vi "TF3710LibExample.vi"() -> ()   [LabVIEW 2020]
uses:
  <userlib>/Beckhoff-LabVIEW-Interface/_DependsOn/TypeDefs/Low-Levels/Symbol Interface Mode.ctl
  <userlib>/Beckhoff-LabVIEW-Interface/_DependsOn/With TypeResolving/Read Sync Single TypeResolved.vi
  <userlib>/Beckhoff-LabVIEW-Interface/_DependsOn/With TypeResolving/Read Async Single TypeResolved.vi
panel:
  out "Read Status? 8":bool
  out "Data 8":variant
  out "Read Status? 7":bool
  out "Data 7":variant
  out "Read Status? 6":bool
  out "Data 6":variant
  out "Read Status? 5":bool
  out "Data 5":variant
  out "Read Status? 4":bool
  out "Data 4":variant
  out "ReadGrpSymbols":string[](array[string])
  out "PortInfo":string
  out "error out":errorcluster
  in  "error in (no error)":errorcluster
  in  "Symbol file path":path=path "C:/MSDApps/GitHub-Projects/EDP Emotor/Anoop_LabviewTwincatADSTesting/ADS Read Symbols.xml"
  out "Read Status?":bool
  out "Read Status? 2":bool
  out "Read Status? 3":bool
  out "Data 1":variant
  out "Data 2":variant
  out "Data 3":variant
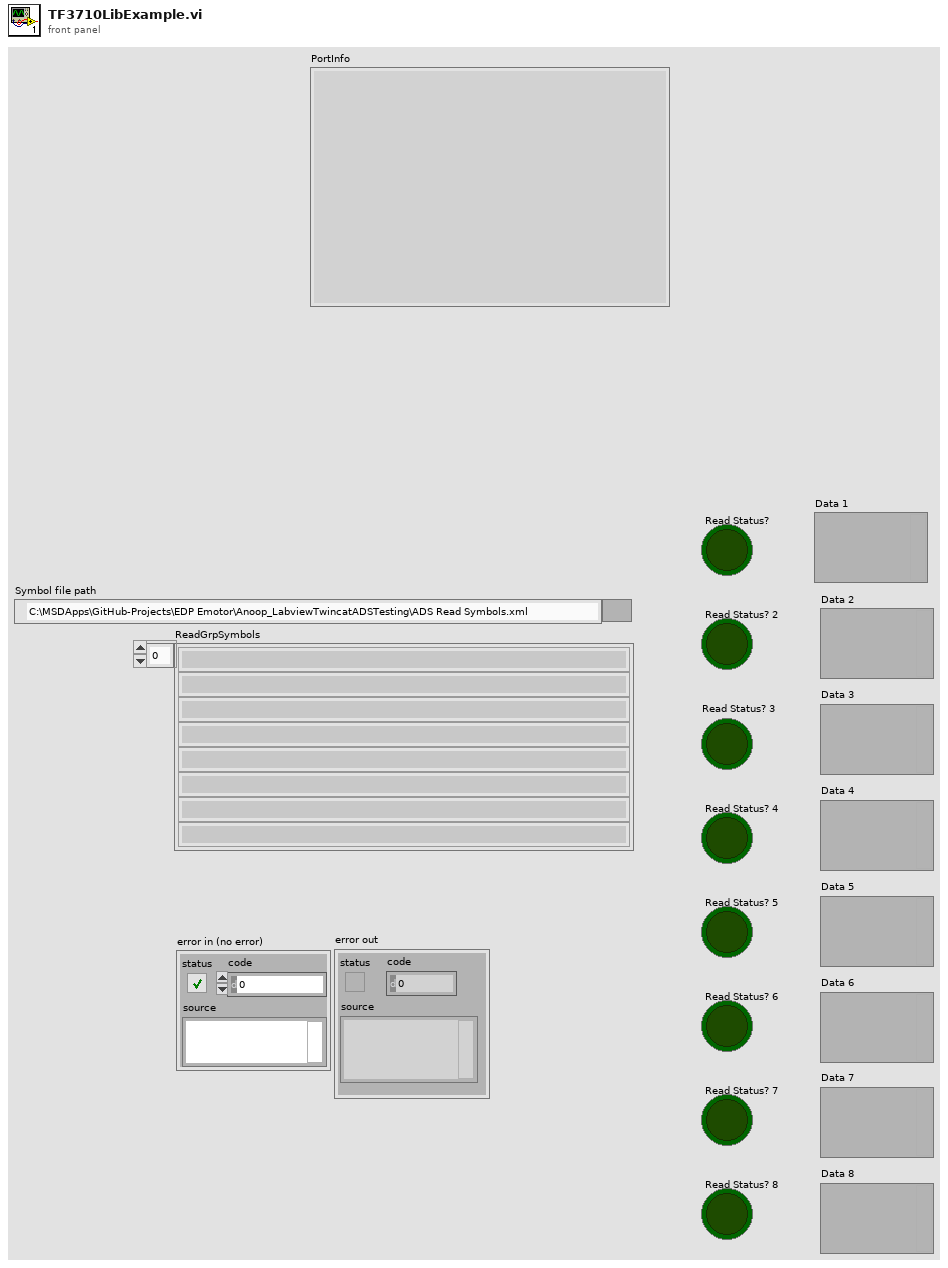
[diagram p1: front panel]
types:
  T1 = typedef "Symbol Interface Mode.ctl" = enum16{"Read Only", "Write Only", "Read & Write"}
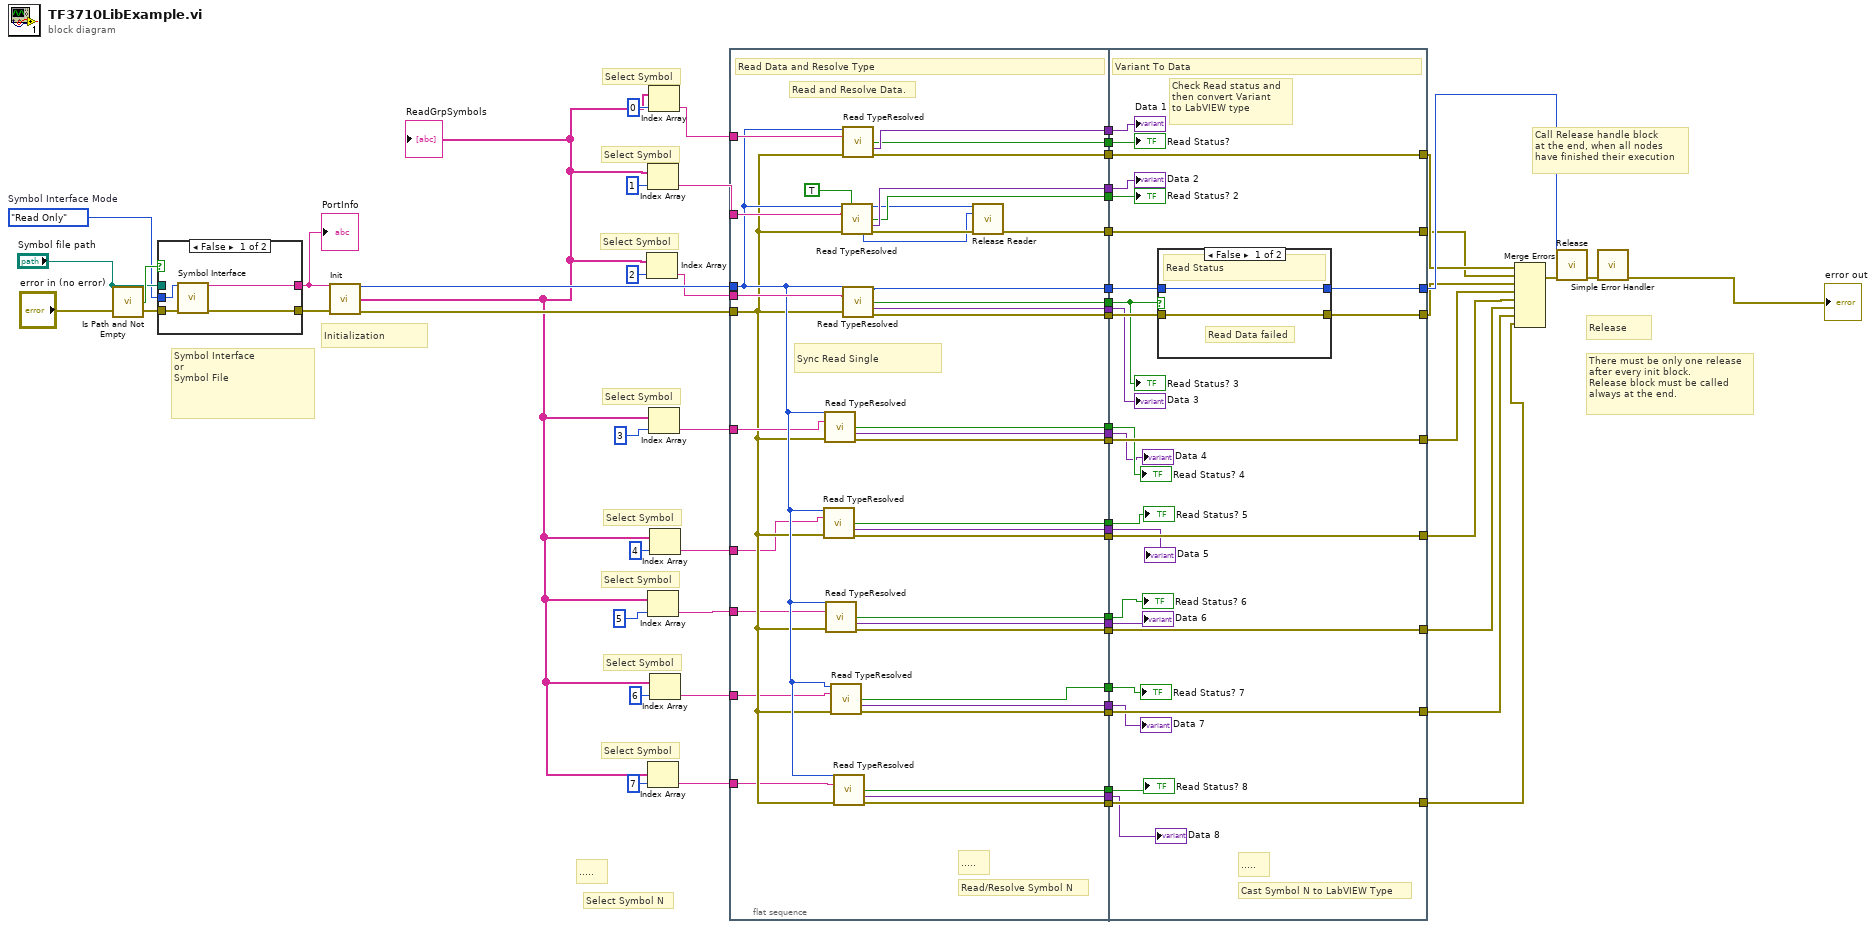
[diagram p0: block diagram]
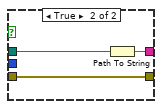
[diagram p2: hidden frame]
diagram:
  w36 = Symbol_Interface_Mode."Read Only"  # Symbol Interface Mode
  # "Select Symbol"
  # "Select Symbol"
  # "Select Symbol"
  # "Select Symbol"
  # "Select Symbol"
  # "Symbol Interface\nor\nSymbol File"
  # "Call Release handle block\nat the end, when all nodes\nhave finished their execution"
  # "Select Symbol N"
  # "....."
  # "Select Symbol"
  # "Select Symbol"
  # "There must be only one release\nafter every init block.\nRelease block must be called\nalways at the end."
  # "Select Symbol"
  # "Initialization"
  # "Release"
  n1 = call <vilib>:"Is Path and Not Empty.vi"("path"="Symbol file path") -> ("Is Path and Not Empty?"=w39:bool)  [unwired: 4 in]
  n2 = case shown="False" w39 {
    tunnel: [w66 w69] -> w32
    tunnel: "Symbol file path" -> [_ w68]
    tunnel: [w65 w67] -> w38
    tunnel: w36 -> [w64 _]
    tunnel: "error in (no error)" -> [w63 w67]
    frame False {
      n3 = call <userlib>:"Symbol Interface.vi"("Symbol Interface Mode"=w64, "error in (no error)"=w63) -> ("PortInfo"=w66:string, "error out"=w65:errorcluster)  [unwired: 12 in]
    }
    frame True {
      n4 = Path To String(path=w68) -> (string=w69:string)
    }
  }
  "PortInfo" <- w32
  n5 = call <userlib>:"Init.vi"("XMLDescription"=w32, "error in (no error)"=w38) -> ("Handle"=w45:u32, "ReadGrpSymbols"=w26:string[], "error out"=w46:errorcluster)  [unwired: 9 in, 2 out]
  "ReadGrpSymbols" <- w26
  n6 = Index Array(array=w26, index=2) -> (element=w44:string)
  n7 = Index Array(array=w26, index=1) -> (element=w48:string)
  n8 = Index Array(array=w26, index=5) -> (element=w4:string)
  n9 = Index Array(array=w26, index=7) -> (element=w2:string)
  n10 = Index Array(array=w26, index=0) -> (element=w47:string)
  n11 = Index Array(array=w26, index=3) -> (element=w25:string)
  n12 = Index Array(array=w26, index=4) -> (element=w5:string)
  n13 = Index Array(array=w26, index=6) -> (element=w3:string)
  n14 = flat-sequence {
    tunnel: w48 -> [w108]
    tunnel: w47 -> [w105]
    tunnel: w46 -> [w89]
    tunnel: w45 -> [w91]
    tunnel: w44 -> [w103]
    tunnel: [w94] -> w62
    tunnel: [w106] -> w61
    tunnel: [w104] -> w60
    tunnel: [w102] -> w59
    tunnel: [w101] -> w58
    tunnel: [w100] -> w57
    tunnel: [w99] -> w56
    tunnel: [w98] -> w55
    tunnel: [w97] -> w54
    tunnel: [w96] -> w53
    tunnel: w25 -> [w90]
    tunnel: [w88] -> w23
    tunnel: [w87] -> w21
    tunnel: [w86] -> w19
    tunnel: [w85] -> w17
    tunnel: [w84] -> w15
    tunnel: [w83] -> w14
    tunnel: [w82] -> w13
    tunnel: [w81] -> w12
    tunnel: [w80] -> w11
    tunnel: [w79] -> w10
    tunnel: [w78] -> w9
    tunnel: [w77] -> w8
    tunnel: [w76] -> w7
    tunnel: [w75] -> w6
    tunnel: w5 -> [w74]
    tunnel: w4 -> [w73]
    tunnel: w3 -> [w72]
    tunnel: w2 -> [w71]
    tunnel: [w70] -> w1
    tunnel: [w130] -> w43
    tunnel: [w132] -> w40
    tunnel: [w135] -> w41
    tunnel: w62 -> [w135]
    tunnel: w61 -> [w134]
    tunnel: w60 -> [w131]
    tunnel: w59 -> [w133]
    tunnel: w58 -> [w126]
    tunnel: w57 -> [w125]
    tunnel: w56 -> [w124]
    tunnel: [w134] -> w42
    tunnel: w55 -> [w127]
    tunnel: w54 -> [w129]
    tunnel: w53 -> [w128]
    tunnel: [w123] -> w24
    tunnel: w23 -> [w123]
    tunnel: [w122] -> w22
    tunnel: w21 -> [w122]
    tunnel: [w121] -> w20
    tunnel: w19 -> [w121]
    tunnel: [w120] -> w18
    tunnel: w17 -> [w120]
    tunnel: [w119] -> w16
    tunnel: w15 -> [w119]
    tunnel: w14 -> [w118]
    tunnel: w13 -> [w117]
    tunnel: w12 -> [w116]
    tunnel: w11 -> [w115]
    tunnel: w10 -> [w114]
    tunnel: w9 -> [w113]
    tunnel: w8 -> [w112]
    tunnel: w7 -> [w111]
    tunnel: w6 -> [w110]
    tunnel: w1 -> [w109]
    frame #0 {
      # "Read and Resolve Data."
      # "Read/Resolve Symbol N"
      # "....."
      # "Sync Read Single"
      # "Read Data and Resolve Type"
      n15 = call-poly <userlib>:"Read TypeResolved.vi"("Handle"=w91, "SymbolName"=w74, "error constant"=w89) -> ("Read Status?"=w82:bool, "RData"=w76:variant, "error out"=w87:errorcluster)  [unwired: 9 in, 1 out]
      n16 = call-poly <userlib>:"Read TypeResolved.vi"("Handle"=w91, "SymbolName"=w90, "error constant"=w89) -> ("Read Status?"=w83:bool, "RData"=w75:variant, "error out"=w88:errorcluster)  [unwired: 9 in, 1 out]
      n17 = call-poly <userlib>:"Read TypeResolved.vi"("Handle"=w91, "SymbolName"=w73, "error constant"=w89) -> ("Read Status?"=w81:bool, "RData"=w70:variant, "error out"=w86:errorcluster)  [unwired: 9 in, 1 out]
      n18 = call-poly <userlib>:"Read TypeResolved.vi"("Handle"=w91, "SymbolName"=w72, "error constant"=w89) -> ("Read Status?"=w80:bool, "RData"=w77:variant, "error out"=w85:errorcluster)  [unwired: 9 in, 1 out]
      n19 = call-poly <userlib>:"Read TypeResolved.vi"("Handle"=w91, "SymbolName"=w71, "error constant"=w89) -> ("Read Status?"=w79:bool, "RData"=w78:variant, "error out"=w84:errorcluster)  [unwired: 9 in, 1 out]
      n20 = call-poly <userlib>:"Read TypeResolved.vi"("Handle"=w91, "Wait?"=TRUE, "SymbolName"=w108, "error constant"=w89) -> ("Handle"=w93:u32, "Read Status?"=w96:bool, "RData"=w100:variant, "ReadHdl"=w92:u32, "error out"=w107:errorcluster)  [unwired: 6 in, 1 out]
      n21 = call-poly <userlib>:"Read TypeResolved.vi"("Handle"=w91, "SymbolName"=w105, "error constant"=w89) -> ("Read Status?"=w97:bool, "RData"=w101:variant, "error out"=w106:errorcluster)  [unwired: 9 in, 1 out]
      n22 = call-poly <userlib>:"Read TypeResolved.vi"("Handle"=w91, "SymbolName"=w103, "error constant"=w89) -> ("Handle"=w102:u32, "Read Status?"=w98:bool, "RData"=w99:variant, "error out"=w104:errorcluster)  [unwired: 9 in]
      n23 = call <userlib>:"Release Reader.vi"("Handle"=w93, "ReadHandle"=w92, "error in (no error)"=w107) -> ("error out"=w94:errorcluster)  [unwired: 11 in, 1 out]
    }
    frame #1 {
      # "Check Read status and\nthen convert Variant \nto LabVIEW type"
      # "Cast Symbol N to LabVIEW Type"
      # "....."
      # "Variant To Data"
      n24 = case shown="False" w127 {
        tunnel: w133 -> [w137 w138]
        tunnel: [w136 w139] -> w132
        tunnel: w131 -> [w136 w139]
        tunnel: [w137 w138] -> w130
        frame False {
          # "Read Data failed"
          # "Read Status"
        }
        frame True {
          # "User Code here"
          # "Variant to Data"
        }
      }
      "Read Status?" <- w129
      "Read Status? 2" <- w128
      "Read Status? 3" <- w127
      "Data 1" <- w126
      "Data 2" <- w125
      "Data 3" <- w124
      "Read Status? 4" <- w118
      "Data 4" <- w110
      "Read Status? 5" <- w117
      "Data 5" <- w111
      "Read Status? 6" <- w116
      "Data 6" <- w109
      "Read Status? 7" <- w115
      "Data 7" <- w112
      "Read Status? 8" <- w114
      "Data 8" <- w113
    }
  }
  n25 = Merge Errors(w42, w41, w40, w24, w22, w20, w18, w16) -> (w52:errorcluster)
  n26 = call <userlib>:"Release.vi"("Handle"=w43, "error in (no error)"=w52) -> ("error out"=w35:errorcluster)  [unwired: 13 in]
  n27 = call <vilib>:"Simple Error Handler.vi"("error in (no error)"=w35) -> ("error out"=→"error out":errorcluster)  [unwired: 4 in, 4 out]
